vi "PAN_DBS_ParseArrays.vi"(6 "full":bool, 7 "name_only":bool, 9 "type":string, 10 "name":string, 11 "Database RefNum in":T1) -> (2 "str out":string)   [LabVIEW 2016]
uses:
  Modules/DBSHAND/private/vis/DatabaseHand_RefNum.ctl
  Modules/DBSHAND/private/vis/DatabaseHand_Element_Get(1DArr).vi
  Modules/DBSHAND/private/vis/DatabaseHand_Element_Get(2DArr).vi
  Modules/DBSHAND/private/vis/DatabaseHand_Element_Get(3DArr).vi
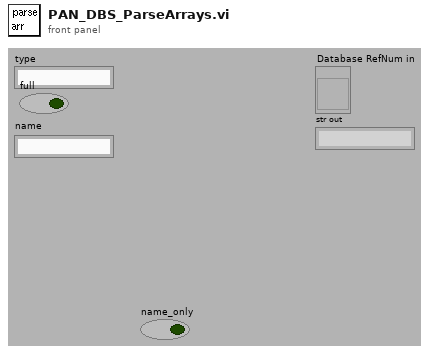
[diagram p1: front panel]
types:
  T1 = typedef "DatabaseHand_RefNum.ctl" = refnum<vi>
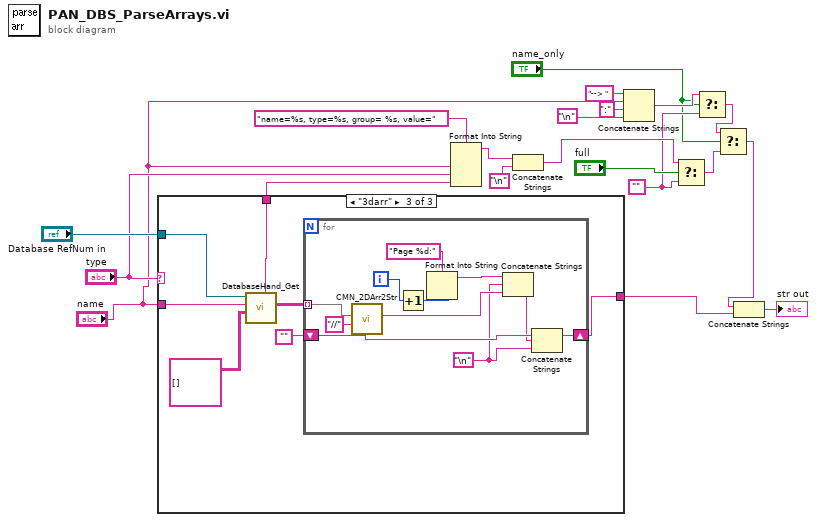
[diagram p0: block diagram]
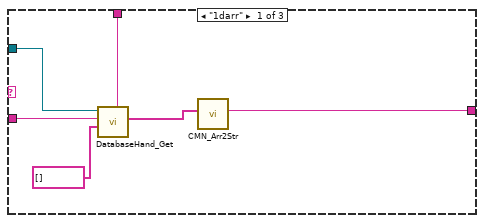
[diagram p2: hidden frame]
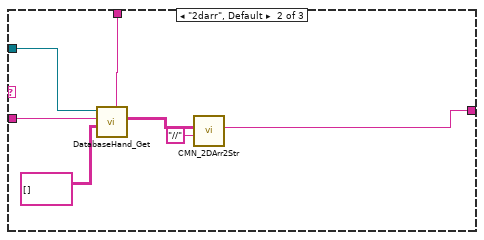
[diagram p3: hidden frame]
diagram:
  w8 = ""
  n1 = case shown="\"3darr\"" "type" {
    tunnel: "Database RefNum in" -> [w26 w32 w39]
    tunnel: "name" -> [w24 w31 w38]
    tunnel: [w22 w28 w34] -> w18
    tunnel: [w21 w33 w40] -> w15
    frame "1darr" {
      n2 = call-poly "DatabaseHand_Get.vi"("default value"=string[] [], "name"=w24, "Database RefNum in"=w26) -> ("value"=w23:string[], "group"=w21:string)  [unwired: 2 in, 5 out]
      n3 = call "CMN_Arr2Str.vi"("Array in"=w23) -> ("string out"=w22:string)  [unwired: 10 out]
    }
    frame "2darr", Default {
      n4 = call-poly "DatabaseHand_Get.vi"("default value"=string[][] [], "name"=w31, "Database RefNum in"=w32) -> ("value"=w29:string[][], "group"=w33:string)  [unwired: 2 in, 5 out]
      n5 = call "CMN_2DArr2Str.vi"("separator"="//", "array in"=w29) -> ("string out"=w28:string)  [unwired: 9 out]
    }
    frame "3darr" {
      n6 = call-poly "DatabaseHand_Get.vi"("default value"=string[][][] [], "name"=w38, "Database RefNum in"=w39) -> ("value"=w36:string[][][], "group"=w40:string)  [unwired: 2 in, 5 out]
      n7 = for {
        tunnel: w36 -> [w50] mode=indexing
        shift-right: [w49] -> w34
        shift-left: "" -> [w48]
        i -> [w46]
        w42 = "\n"
        n8 = call "CMN_2DArr2Str.vi"("separator"="//", "array in"=w50) -> ("string out"=w43:string)  [unwired: 9 out]
        n9 = Increment(x=w46) -> (x+1=w45:i32)
        n10 = Format Into String(format string="Page %d:", w45) -> (resulting string=w44:string)  [unwired: 2 in, 1 out]
        n11 = Concatenate Strings(w44, w42, w43) -> (w41:string)
        n12 = Concatenate Strings(w48, w41, w42) -> (w49:string)
      }
    }
  }
  n13 = Format Into String(format string="name=%s, type=%s, group= %s, value=", "name", "type", w15) -> (resulting string=w14:string)  [unwired: 2 in, 1 out]
  n14 = Concatenate Strings(w14, "\n") -> (w12:string)
  n15 = Concatenate Strings("--> " ("string"), "name", ":" ("string"), "\n") -> (w9:string)
  n16 = Select(t=w12, s="full", f=w8) -> (s? t:f=w6:string)
  n17 = Select(t=w9, s="name_only", f=w8) -> (s? t:f=w7:string)
  n18 = Select(t=w7, s="name_only", f=w6) -> (s? t:f=w5:string)
  n19 = Concatenate Strings(w5, w18) -> (→"str out":string)
